vi "Set Signal Viewer.vi"(5 "Trigger Level Reference":refnum<vi>, 7 "Signal Viewer Reference":refnum<vi>, 8 "Error in":errorcluster, 11 "State Variables in":T1={"Stop Notifier"=refnum, "UI References"=[], "DAQmx"={"ECG Input"={"Channel"="", "Task"="", "Max Value"=0.0, "Min Value"=0.0, "Sampling Rate"=0.0, "Batch Size"=0}, "Trigger Output"={"Channel"="", "Task"="", "Pulse Frequency"=0.0, "Delay"=0, "Triggers per Shot"=0}}, "Data Queue"=refnum, "Filter"={"Batch Size"=1000, "Update Cycle"=0, "Filter Buffer"=[]}, "Last Detect Result"=FALSE}) -> (0 "Error out":errorcluster, 3 "State Variables out":T1={"Stop Notifier"=refnum, "UI References"=[], "DAQmx"={"ECG Input"={"Channel"="", "Task"="", "Max Value"=0.0, "Min Value"=0.0, "Sampling Rate"=0.0, "Batch Size"=0}, "Trigger Output"={"Channel"="", "Task"="", "Pulse Frequency"=0.0, "Delay"=0, "Triggers per Shot"=0}}, "Data Queue"=refnum, "Filter"={"Batch Size"=1000, "Update Cycle"=0, "Filter Buffer"=[]}, "Last Detect Result"=FALSE})   [LabVIEW 2014, in "Flow Control.lvlib"]
uses:
  Flow Control.lvlib
  Controls/State Variables.ctl
  Controls/DAQmx Variables.ctl
  Controls/Filter Variables.ctl
  <vilib>/Utility/miscctls.llb/LVRangeTypeDef.ctl
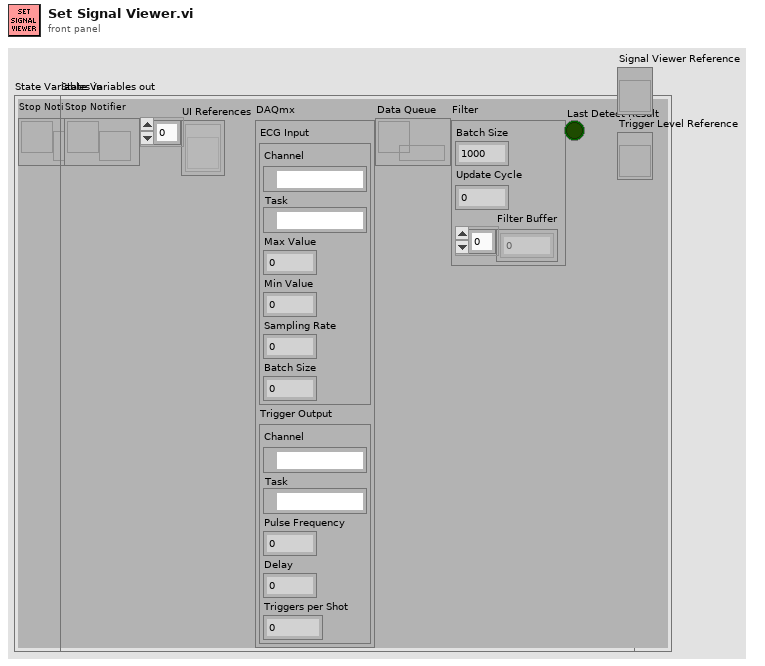
[diagram p1: front panel]
types:
  T1 = typedef "State Variables.ctl" = cluster{"Stop Notifier":refnum<notifier>, "UI References":refnum<vi>[], "DAQmx":T2, "Data Queue":refnum<queue>, "Filter":T3, "Last Detect Result":bool}
  T2 = typedef "DAQmx Variables.ctl" = cluster{"ECG Input":cluster{"Channel":tag, "Task":refnum<k21>, "Max Value":dbl, "Min Value":dbl, "Sampling Rate":dbl, "Batch Size":i32}, "Trigger Output":cluster{"Channel":tag, "Task":refnum<k21>, "Pulse Frequency":dbl, "Delay":u16, "Triggers per Shot":i32}}
  T3 = typedef "Filter Variables.ctl" = cluster{"Batch Size":i32, "Update Cycle":i32, "Filter Buffer":dbl[]}
  T4 = typedef "LVRangeTypeDef.ctl" = cluster{"Minimum":dbl, "Maximum":dbl, "Increment":dbl, "Minor Increment":dbl, "Start":dbl}
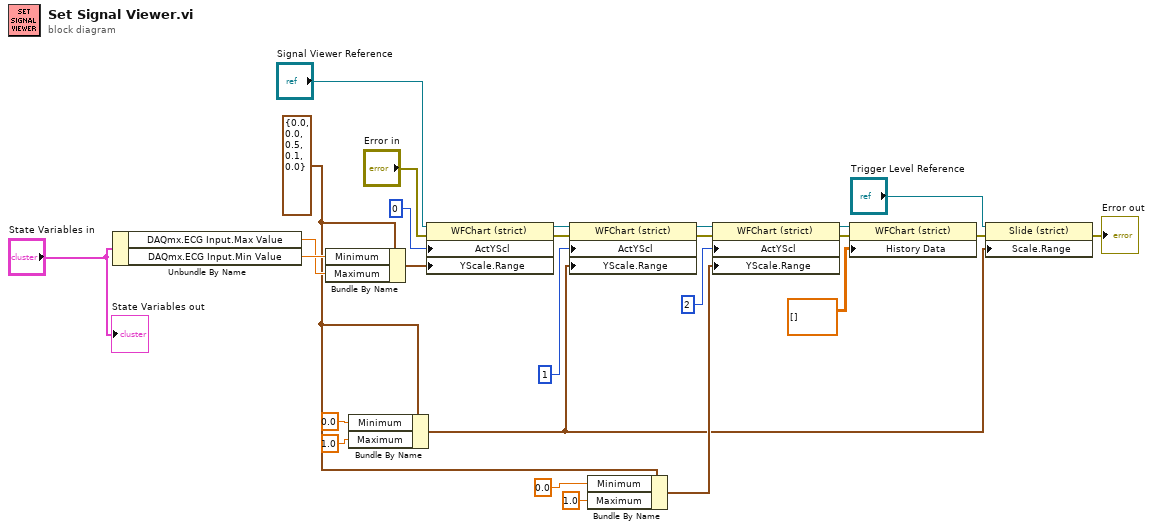
[diagram p0: block diagram]
diagram:
  w9 = T4 {"Minimum"=0.0, "Maximum"=0.0, "Increment"=0.5, "Minor Increment"=0.1, "Start"=0.0} ("Y Scale.Range")
  n1 = Unbundle By Name("State Variables in") -> ("DAQmx.ECG Input.Max Value"=w18:dbl, "DAQmx.ECG Input.Min Value"=w19:dbl)
  n2 = Bundle By Name(cluster=w9, "Minimum"=w19, "Maximum"=w18) -> (w20:T4)
  n3 = Bundle By Name(cluster=w9, "Minimum"=0.0, "Maximum"=1.0) -> (w6:T4)
  n4 = property on="Property Node" class="WFChart (strict)"(reference="Signal Viewer Reference", error in="Error in", "ActYScl"=0 ("Active Y Scale"), "YScale.Range"=w20) -> (reference out=w17:refnum<vi>, error out=w14:errorcluster)
  n5 = property on="Property Node" class="WFChart (strict)"(reference=w17, error in=w14, "ActYScl"=1 ("Active Y Scale"), "YScale.Range"=w6) -> (reference out=w16:refnum<vi>, error out=w13:errorcluster)
  n6 = Bundle By Name(cluster=w9, "Minimum"=0.0, "Maximum"=1.0) -> (w8:T4)
  n7 = property on="Property Node" class="WFChart (strict)"(reference=w16, error in=w13, "ActYScl"=2 ("Active Y Scale"), "YScale.Range"=w8) -> (reference out=w4:refnum<vi>, error out=w3:errorcluster)
  n8 = property on="Property Node" class="WFChart (strict)"(reference=w4, error in=w3, "History Data"=dbl[][] [] ("Signal Viewer")) -> (error out=w2:errorcluster)  [unwired: 1 out]
  n9 = property on="Property Node" class="Slide (strict)"(reference="Trigger Level Reference", error in=w2, "Scale.Range"=w6) -> (error out=→"Error out":errorcluster)  [unwired: 1 out]
  "State Variables out" <- "State Variables in"
